vi "Get Owning Task.vi"(8 "error in (no error)":errorcluster, 11 "GroupAbstract in":refnum<class "GroupAbstract.lvclass">) -> (0 "error out":errorcluster, 2 "Task":string, 3 "GroupAbstract out":refnum<class "GroupAbstract.lvclass">)   [LabVIEW 2020, in "Vecto.lvlib" / "GroupAbstract.lvclass"]
uses:
  GroupAbstract.lvclass
  GroupAbstract.lvclass/GroupAbstract.ctl
  Group Config/Group Config.lvclass
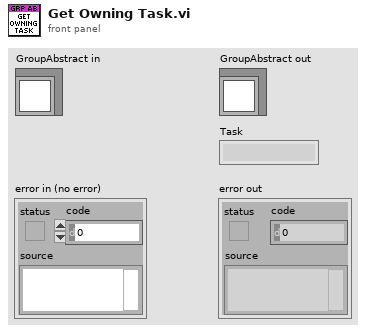
[diagram p1: front panel]
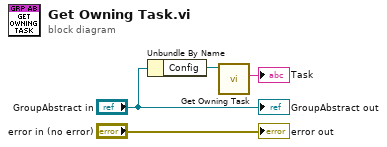
[diagram p0: block diagram]
diagram:
  n1 = Unbundle By Name("GroupAbstract in") -> ("Config"=w2:refnum<class "Group Config.lvclass">)
  n2 = call "Get Owning Task.vi"("Group Config in"=w2) -> ("Task"=→"Task":string)  [unwired: 8 in, 2 out]
  "error out" <- "error in (no error)"
  "GroupAbstract out" <- "GroupAbstract in"
